vi "ExampleScript.vi"   [LabVIEW 2016, in "Script.lvlib"]
uses:
  Script.lvlib
  <vilib>/Wiresmith Technology/G CLI/Argument Parser/Option Class/Option Configuration.ctl
  <vilib>/Wiresmith Technology/G CLI/Argument Parser/Option Class/Argument Type.ctl
  <vilib>/Wiresmith Technology/G CLI/CLI Class/CLI.lvclass
  <vilib>/Wiresmith Technology/G CLI/Argument Parser/Option Class/Option.lvclass
  <vilib>/Wiresmith Technology/G CLI/Argument Parser/Option Set Class/Option Set.lvclass
types:
  T1 = typedef "Option Parser.lvlib/Option.lvclass/Option Configuration.ctl" = cluster{"Option Type":T2, "Option Labels":string[], "Key":string, "Description":string, "Required":bool, "Default Value":string}
  T2 = typedef "Option Parser.lvlib/Option.lvclass/Argument Type.ctl" = enum16{"flag", "value"}
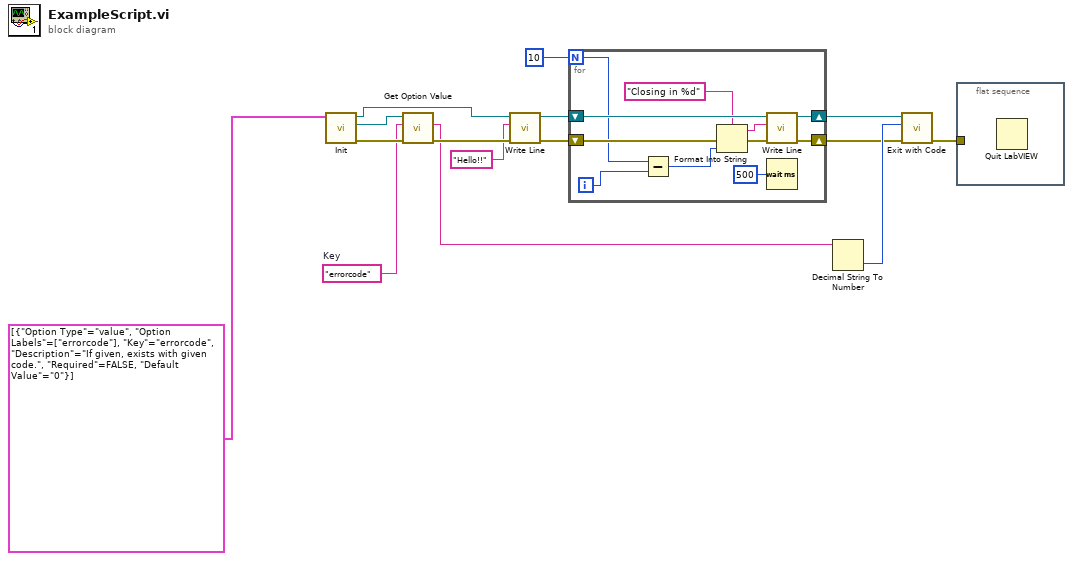
[diagram p0: block diagram]
diagram:
  w9 = "errorcode"  # Key
  n1 = call "Init.vi"("Options"=T1[] [{"Option Type"=enum."value", "Option Labels"=["errorcode"], "Key"="errorcode", "Description"="If given, exists with given code.", "Required"=FALSE, "Default Value"="0"}]) -> ("error out"=w13:errorcluster, "Option Set out"=w11:refnum<class "Option Set.lvclass">, "CLI out"=w15:refnum<class "CLI.lvclass">)  [unwired: 8 in]
  n2 = call <vilib>:"Get Option Value.vi"("error in (no error)"=w13, "Option Key"=w9, "Option Set in"=w11) -> ("error out"=w12:errorcluster, "Value"=w7:string)  [unwired: 5 in, 2 out]
  n3 = call <vilib>:"Write Line.vi"("error in (no error)"=w12, "Text to Write"="Hello!!", "CLI in"=w15) -> ("error out"=w2:errorcluster, "CLI out"=w5:refnum<class "CLI.lvclass">)  [unwired: 7 in]
  n4 = for {
    N: 10 -> [w18]
    shift-right: [w25] -> w4
    shift-left: w5 -> [w26]
    shift-right: [w24] -> w3
    shift-left: w2 -> [w23]
    i -> [w17]
    n5 = Subtract(x=w18, y=w17) -> (x-y=w16:i32)
    n6 = Format Into String(format string="Closing in %d" ("Text to Write"), error in=w23, w16) -> (resulting string=w19:string, error out=w21:errorcluster)  [unwired: 1 in]
    n7 = call <vilib>:"Write Line.vi"("error in (no error)"=w21, "Text to Write"=w19, "CLI in"=w26) -> ("error out"=w24:errorcluster, "CLI out"=w25:refnum<class "CLI.lvclass">)  [unwired: 7 in]
    n8 = Wait (ms)(milliseconds to wait=u32 500) -> ()  [unwired: 1 out]
  }
  n9 = Decimal String To Number(string=w7) -> (number=w8:i32)  [unwired: 2 in, 1 out]
  n10 = call <vilib>:"Exit with Code.vi"("error in (no error)"=w3, "Exit Code (0)"=w8, "CLI in"=w4) -> ("error out"=w6:errorcluster)  [unwired: 8 in]
  n11 = flat-sequence {
    tunnel: w6 -> [_]
    frame #0 {
      n12 = Quit LabVIEW() -> ()  [unwired: 1 in]
    }
  }
